vi "ZDataVIS_XY_Offset+Mult.vi"(7 "Voffset -2T":dbl, 8 "error in (no error)":errorcluster, 10 "X Step Info":cluster{"X Low":dbl, "X High":dbl, "X Step":dbl}={"X Low"=-0.1, "X High"=0.1, "X Step"=4e-05} {"X Step" format="%#_6p"; "X High" format="%#_6p"; "X Low" format="%#_6p"}, 11 "State Wire IN":T1={"Core"={"Current VI Reference"=refnum, "Close Panel on Exit?"=FALSE}, "Sweep Data Cluster"={"Vfast"=[], "Vslow"=[], "Vslowest"=[], "Comments"="", "Scan names"=[]}, "Cursor Info"={"Fast Index"=[], "Slow Index"=0.0, "Slow Indices"=[], "Raw Cursor Position"={"X"=0.0, "Y"=0.0}, "Field / temp"=0}, "Scan names"=[], "Data DVR"=refnum, "Arr of Y arrays (intensity info)"=[], "Decimated X values"=[], "X Step Info"={"X Low"=-0.1, "X High"=0.1, "X Step"=4e-05}, "Voffset -2T"=0.0} {"X Step Info"."X Step" format="%#_6p"; "X Step Info"."X High" format="%#_6p"; "X Step Info"."X Low" format="%#_6p"}) -> (0 "error out":errorcluster, 1 "Y Offset+Mult":cluster{"Offset X Low":dbl, "X Step":dbl}, 2 "X Offset+Mult":cluster{"Offset X Low":dbl, "X Step":dbl}, 3 "State Wire OUT":T1={"Core"={"Current VI Reference"=refnum, "Close Panel on Exit?"=FALSE}, "Sweep Data Cluster"={"Vfast"=[], "Vslow"=[], "Vslowest"=[], "Comments"="", "Scan names"=[]}, "Cursor Info"={"Fast Index"=[], "Slow Index"=0.0, "Slow Indices"=[], "Raw Cursor Position"={"X"=0.0, "Y"=0.0}, "Field / temp"=0}, "Scan names"=[], "Data DVR"=refnum, "Arr of Y arrays (intensity info)"=[], "Decimated X values"=[], "X Step Info"={"X Low"=-0.1, "X High"=0.1, "X Step"=4e-05}, "Voffset -2T"=0.0} {"X Step Info"."X Step" format="%#_6p"; "X Step Info"."X High" format="%#_6p"; "X Step Info"."X Low" format="%#_6p"})   [LabVIEW 2016]
uses:
  ZDataVIS_StateWire.ctl
  <vilib>/Utility/miscctls.llb/LVPointDoubleTypeDef.ctl
panel:
  # "cursor x"
  # "cursor y"
  # "cursor x"
  # "cursor y"
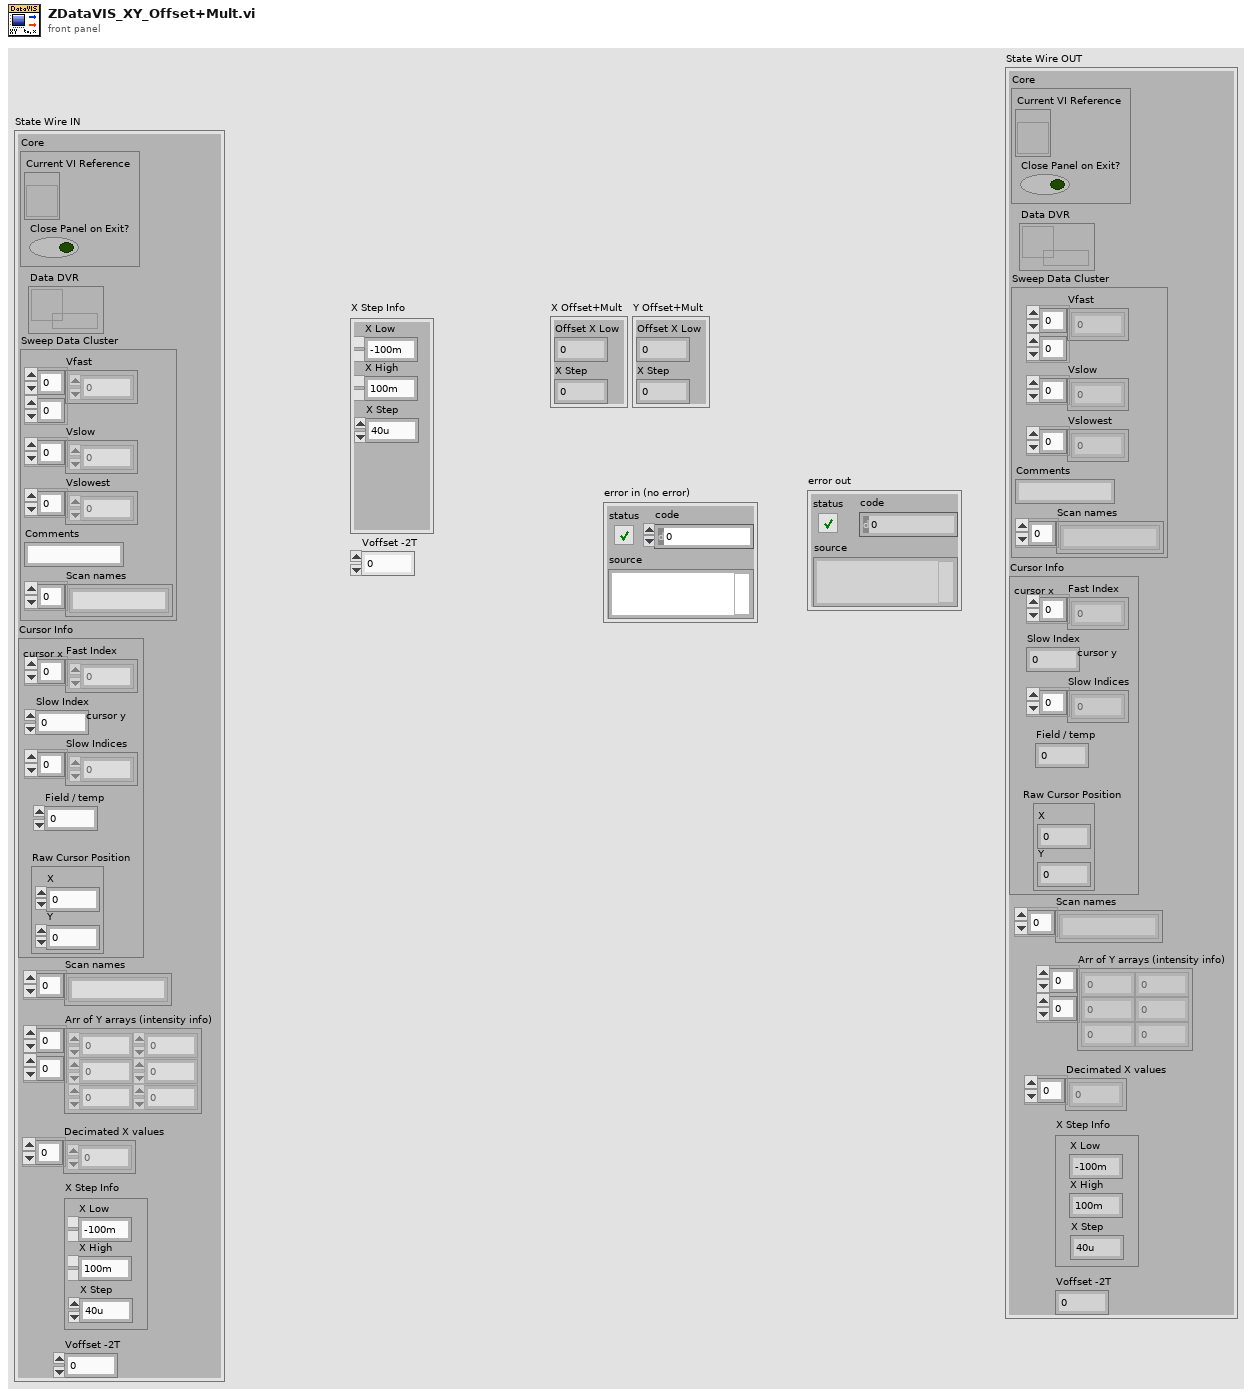
[diagram p1: front panel]
types:
  T1 = typedef "ZDataVIS_StateWire.ctl" = cluster{"Core":cluster{"Current VI Reference":refnum<vi>, "Close Panel on Exit?":bool}, "Sweep Data Cluster":cluster{"Vfast":dbl[][], "Vslow":dbl[], "Vslowest":dbl[], "Comments":string, "Scan names":string[]}, "Cursor Info":cluster{"Fast Index":dbl[], "Slow Index":dbl, "Slow Indices":dbl[], "Raw Cursor Position":T2, "Field / temp":i32}, "Scan names":string[], "Data DVR":refnum<data-value>, "Arr of Y arrays (intensity info)":dbl[][], "Decimated X values":dbl[], "X Step Info":cluster{"X Low":dbl, "X High":dbl, "X Step":dbl}, "Voffset -2T":dbl}
  T2 = typedef "LVPointDoubleTypeDef.ctl" = cluster{"X":dbl, "Y":dbl}
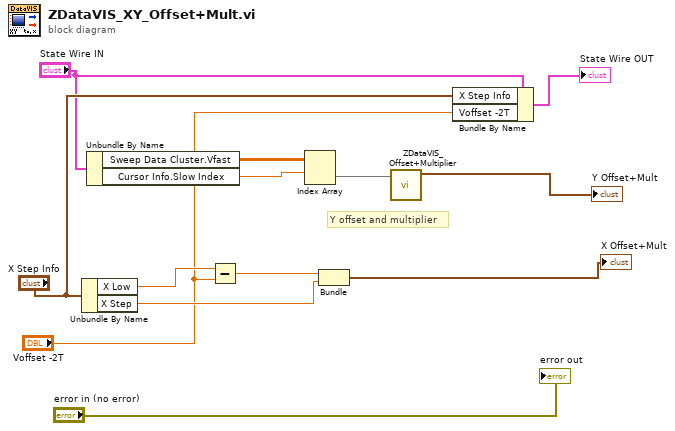
[diagram p0: block diagram]
diagram:
  # "Y offset and multiplier"
  n1 = Unbundle By Name("X Step Info") -> ("X Low"=w8:dbl, "X Step"=w9:dbl)
  n2 = Unbundle By Name("State Wire IN") -> ("Sweep Data Cluster.Vfast"=w12:dbl[][], "Cursor Info.Slow Index"=w11:dbl)
  n3 = Subtract(x=w8, y="Voffset -2T") -> (x-y=w7:dbl)
  n4 = Index Array(array=w12, index (row)=w11) -> (element=w13:dbl[])  [unwired: 1 in]
  n5 = Bundle(w7, "X Step"=w9) -> (→"X Offset+Mult":cluster{dbl, "X Step":dbl})  [unwired: 1 in]
  n6 = call "ZDataVIS_Offset+Multiplier.vi"("Vfast"=w13) -> ("Cluster"=→"Y Offset+Mult":cluster{dbl, dbl})  [unwired: 10 in]
  n7 = Bundle By Name(cluster="State Wire IN", "X Step Info"="X Step Info", "Voffset -2T"="Voffset -2T") -> (→"State Wire OUT":T1)
  "error out" <- "error in (no error)"
